vi "Instrument_Comm_Main.vi"(8 "error in (no error)":errorcluster) -> (0 "error out":errorcluster)   [LabVIEW 2019, in "Service.lvlib"]
uses:
  Service.lvlib
  MsgQ/MsgQ.lvlib
  <vilib>/Field R&D Services/Logger/Field_RnD_Services_Logger_Toolkit.lvlib
  <vilib>/Field R&D Services/Logger/Type Definitions/Severity.ctl
  <vilib>/addons/zeromq/zmq_context.lvclass
  <vilib>/addons/zeromq/zmq_socket.lvclass
  <vilib>/addons/zeromq/socket_type.ctl
  <vilib>/addons/zeromq/zeromq.lvlib
  <vilib>/addons/zeromq/socket_options.ctl
  mmw_command_lib/src_LabVIEW/mmW_commands/mmW_commands.lvlib
panel:
  out "reply":string
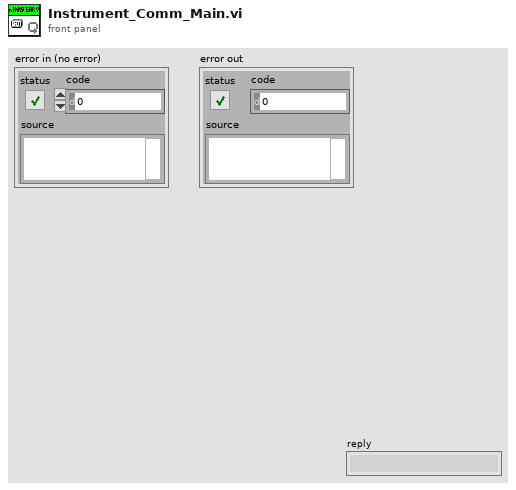
[diagram p1: front panel]
types:
  T1 = typedef "zeromq.lvlib/socket_options.ctl" = enum8{"NONE", "ZMQ_HWM", "<2>", "ZMQ_SWAP", "ZMQ_AFFINITY", "ZMQ_IDENTITY", "ZMQ_SUBSCRIBE", "ZMQ_UNSUBSCRIBE", "ZMQ_RATE", "ZMQ_RECOVERY_IVL", "ZMQ_MCAST_LOOP", "ZMQ_SNDBUF", "ZMQ_RCVBUF", "ZMQ_RCVMORE", "ZMQ_FD", "ZMQ_EVENTS", "ZMQ_TYPE", "ZMQ_LINGER", "ZMQ_RECONNECT_IVL", "ZMQ_BACKLOG", "ZMQ_RECOVERY_IVL_MSEC", "ZMQ_RECONNECT_IVL_MAX", "ZMQ_MAXMSGSIZE", "ZMQ_SNDHWM", "ZMQ_RCVHWM", "ZMQ_MULTICAST_HOPS", "<26>", "ZMQ_RCVTIMEO", "ZMQ_SNDTIMEO", "<29>", "<30>", "ZMQ_IPV4ONLY", "ZMQ_LAST_ENDPOINT", "ZMQ_ROUTER_MANDATORY", "ZMQ_TCP_KEEPALIVE", "ZMQ_TCP_KEEPALIVE_CNT", "ZMQ_TCP_KEEPALIVE_IDLE", "ZMQ_TCP_KEEPALIVE_INTVL", "ZMQ_TCP_ACCEPT_FILTER", "ZMQ_DELAY_ATTACH_ON_CONNECT", "ZMQ_XPUB_VERBOSE"}
  T2 = typedef "zeromq.lvlib/socket_type.ctl" = enum8{"ZMQ_PAIR", "ZMQ_PUB", "ZMQ_SUB", "ZMQ_REQ", "ZMQ_REP", "ZMQ_DEALER", "ZMQ_ROUTER", "ZMQ_PULL", "ZMQ_PUSH", "ZMQ_XPUB", "ZMQ_XSUB"}
  T3 = typedef "Field_RnD_Services_Logger_Toolkit.lvlib/Severity.ctl" = enum16{"Benign", "Warning", "Recoverable", "Fatal"}
  T4 = typedef "Service.lvlib/AppData.ctl" = cluster{"MsgQ":refnum<queue>, "Stop?":bool, "zmq sessions":cluster{"Control_endpoint":string, "Instr_endpoint":string}, "control-loop":cluster{"fromUI-Q":refnum<queue>, "toUI":refnum<user-event>, "Control_endpoint":string}, "UI-loop":cluster{"evnt_ref":refnum<event-registration>}, "logging":cluster{"level":dbl, "verbosity":dbl, "path":string, "Listener_ID":string}}
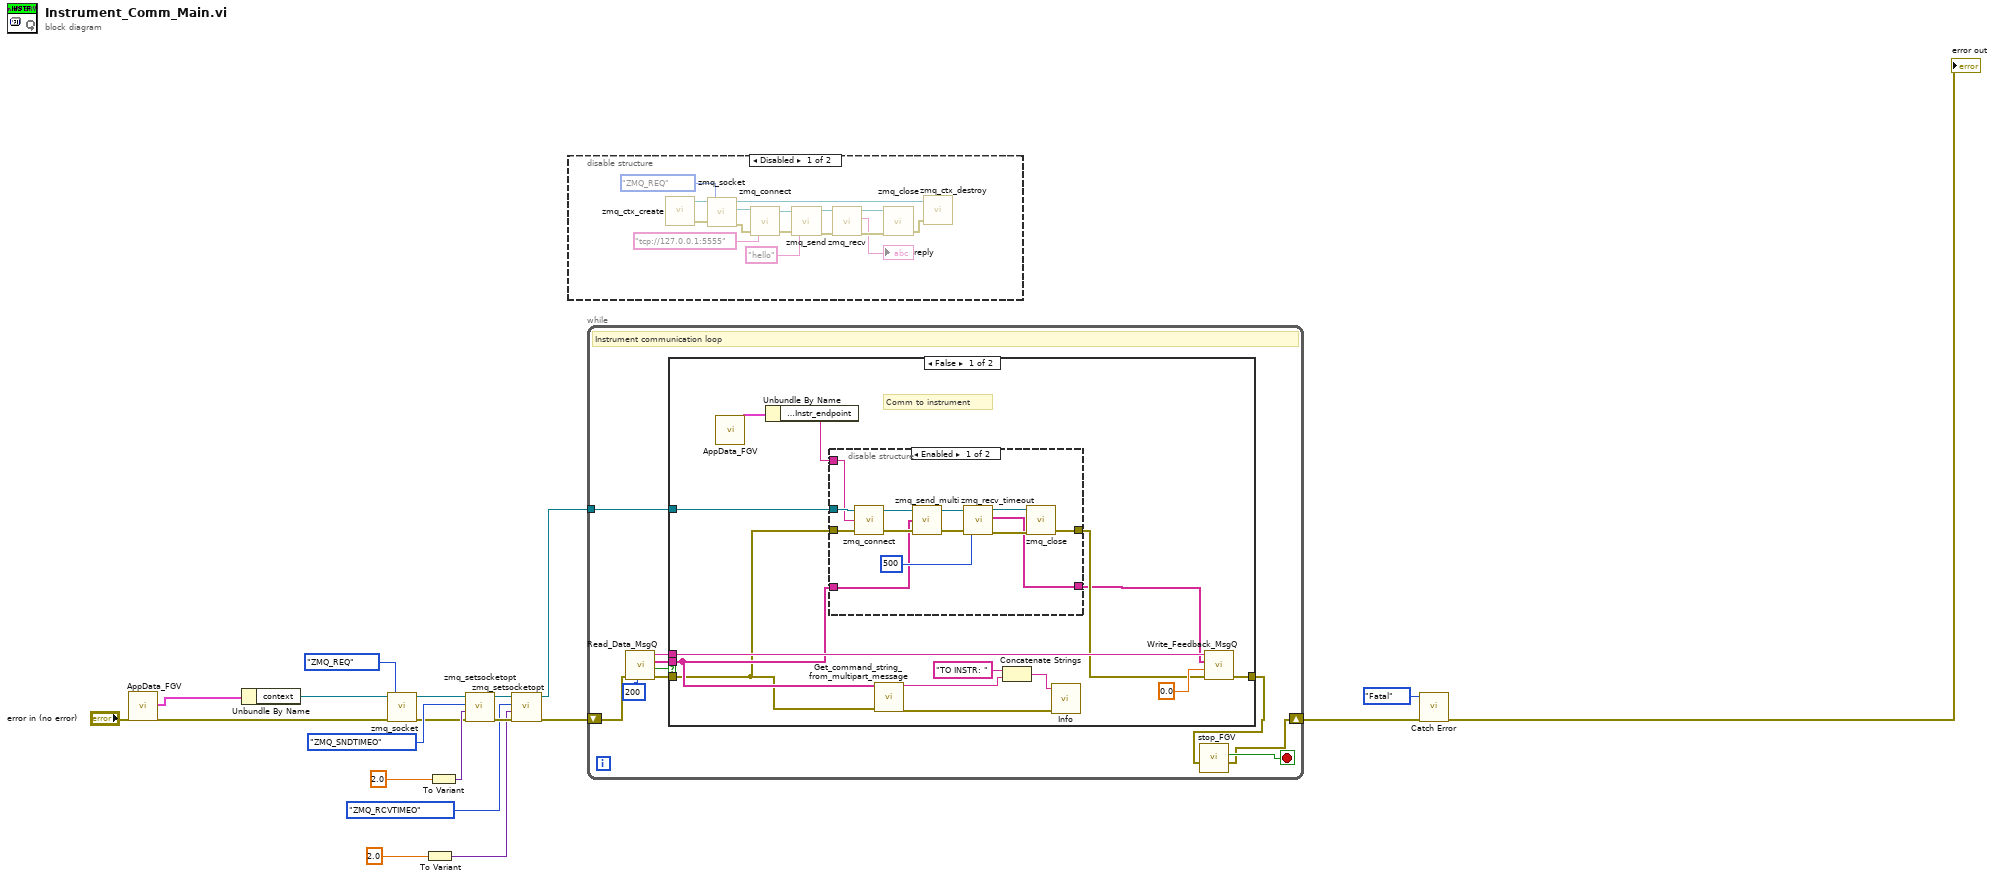
[diagram p0: block diagram]
diagram:
  n1 = call "AppData_FGV.vi"("error in (no error)"="error in (no error)") -> ("AppData out"=w16:T4, "error out"=w4:errorcluster)  [unwired: 17 in]
  n2 = Unbundle By Name(w16) -> ("context"=w2:refnum<class "zmq_context.lvclass">)
  n3 = call <vilib>:"zmq_socket.vi"("error in"=w4, "socket type"=socket_type."ZMQ_REQ", "context in"=w2) -> ("error out"=w10:errorcluster, "socket out"=w14:refnum<class "zmq_socket.lvclass">)  [unwired: 2 in, 1 out]
  n4 = To Variant(anything=2.0) -> (Variant=w5:variant)
  n5 = To Variant(anything=2.0) -> (Variant=w12:variant)
  n6 = call <vilib>:"zmq_setsocketopt.vi"("error in"=w10, "value"=w12, "option"=socket_options."ZMQ_SNDTIMEO", "socket in"=w14) -> ("error out"=w8:errorcluster, "socket out"=w9:refnum<class "zmq_socket.lvclass">)  [unwired: 2 in]
  n7 = call <vilib>:"zmq_setsocketopt.vi"("error in"=w8, "value"=w5, "option"=socket_options."ZMQ_RCVTIMEO", "socket in"=w9) -> ("error out"=w3:errorcluster, "socket out"=w1:refnum<class "zmq_socket.lvclass">)  [unwired: 2 in]
  n8 = disable-structure shown="Disabled" {
    frame Disabled {
      n9 = call <vilib>:"zmq_ctx_create.vi"() -> ("error out"=w26:errorcluster, "context out"=w36:refnum<class "zmq_context.lvclass">)  [unwired: 4 in]
      n10 = call <vilib>:"zmq_socket.vi"("error in"=w26, "socket type"=socket_type."ZMQ_REQ", "context in"=w36) -> ("error out"=w35:errorcluster, "socket out"=w34:refnum<class "zmq_socket.lvclass">, "context out"=w27:refnum<class "zmq_context.lvclass">)  [unwired: 2 in]
      n11 = call <vilib>:"zmq_connect.vi"("error in"=w35, "endpoint"="tcp://127.0.0.1:5555", "socket in"=w34) -> ("error out"=w33:errorcluster, "socket out"=w32:refnum<class "zmq_socket.lvclass">)  [unwired: 1 in]
      n12 = call <vilib>:"zmq_send.vi"("error in"=w33, "data"="hello", "socket in"=w32) -> ("error out"=w25:errorcluster, "socket out"=w31:refnum<class "zmq_socket.lvclass">)  [unwired: 4 in]
      n13 = call <vilib>:"zmq_recv.vi"("error in"=w25, "socket in"=w31) -> ("error out"=w30:errorcluster, "data"=→"reply":string, "socket out"=w29:refnum<class "zmq_socket.lvclass">)  [unwired: 3 in, 2 out]
      n14 = call <vilib>:"zmq_close.vi"("error in"=w30, "socket"=w29) -> ("error out"=w28:errorcluster)  [unwired: 3 in]
      n15 = call <vilib>:"zmq_ctx_destroy.vi"("error in"=w28, "context in"=w27) -> ()  [unwired: 3 in, 1 out]
    }
    frame Enabled {
    }
  }
  n16 = while {
    shift-right: [w38] -> w20
    shift-left: w3 -> [w46]
    tunnel: w1 -> [w37]
    stop <- w40 stop-if-true
    # "Instrument communication loop"
    n17 = call "Read_Data_MsgQ.vi"("timeout in ms (10)"=200, "error in (no error)"=w46) -> ("error out"=w43:errorcluster, "timed out?"=w44:bool, "Data out"=w42:string[], "ResponseAddr"=w41:string)  [unwired: 5 in, 1 out]
    n18 = case shown="False" w44 {
      tunnel: w43 -> [w51 w76]
      tunnel: w42 -> [w52 _]
      tunnel: w41 -> [w60 _]
      tunnel: [w59 w76] -> w39
      tunnel: w37 -> [w56 _]
      frame False {
        # "Comm to instrument"
        n19 = call "AppData_FGV.vi"() -> ("AppData out"=w54:T4)  [unwired: 18 in, 1 out]
        n20 = Unbundle By Name(w54) -> ("zmq sessions.Instr_endpoint"=w53:string)
        n21 = disable-structure shown="Enabled" {
          disable-tunnel: w56 -> [w73 _]
          disable-tunnel: [w72 w75] -> w57
          disable-tunnel: w51 -> [w71 w75]
          disable-tunnel: w53 -> [w62 w74]
          disable-tunnel: [w63 w74] -> w55
          disable-tunnel: w52 -> [w61 _]
          frame Enabled {
            n22 = call <vilib>:"zmq_connect.vi"("error in"=w71, "endpoint"=w62, "socket in"=w73) -> ("error out"=w69:errorcluster, "socket out"=w70:refnum<class "zmq_socket.lvclass">)  [unwired: 1 in]
            n23 = call <vilib>:"zmq_send_multi.vi"("error in"=w69, "parts"=w61, "socket in"=w70) -> ("error out"=w67:errorcluster, "socket out"=w68:refnum<class "zmq_socket.lvclass">)  [unwired: 1 in]
            n24 = call <vilib>:"zmq_recv_timeout.vi"("error in"=w67, "timeout (ms)"=u32 500, "socket in"=w68) -> ("error out"=w65:errorcluster, "parts"=w63:string[], "socket out"=w64:refnum<class "zmq_socket.lvclass">)  [unwired: 1 in, 1 out]
            n25 = call <vilib>:"zmq_close.vi"("error in"=w65, "socket"=w64) -> ("error out"=w72:errorcluster)  [unwired: 3 in]
          }
          frame Disabled {
          }
        }
        n26 = call "Get_command_string_from_multipart_message.vi"("Multipart message in"=w52, "error in (no error)"=w51) -> ("command string out"=w49:string, "error out"=w50:errorcluster)  [unwired: 12 in]
        n27 = Concatenate Strings("TO INSTR: " ("string"), w49) -> (w47:string)
        n28 = call <vilib>:"Info.vi"("Error In"=w50, "Message"=w47) -> ()  [unwired: 9 in, 1 out]
        n29 = call "Write_Feedback_MsgQ.vi"("error in (no error)"=w57, "Code"=0.0, "Data in"=w55, "ResponseAddr"=w60) -> ("error out"=w59:errorcluster)  [unwired: 7 in]
      }
      frame True {
      }
    }
    n30 = call "stop_FGV"("error in (no error)"=w39) -> ("error out"=w38:errorcluster, "stop?"=w40:bool)  [unwired: 7 in]
  }
  n31 = call <vilib>:"Catch Error.vi"("Error In"=w20, "Severity"=Severity."Fatal") -> ("Error Out"=→"error out":errorcluster)  [unwired: 9 in]
